vi "TensorFLow.vi"(8 "error in (no error)":errorcluster, 11 "TFinfo In":T1) -> (0 "Label":string, 1 "Percentages":u8[](array[slide]) scale=0.0..100.0, 2 "Fits":dbl[][](array[numeric]), 3 "TFinfo out":T1, 5 "Labels":string)   [LabVIEW 2019]
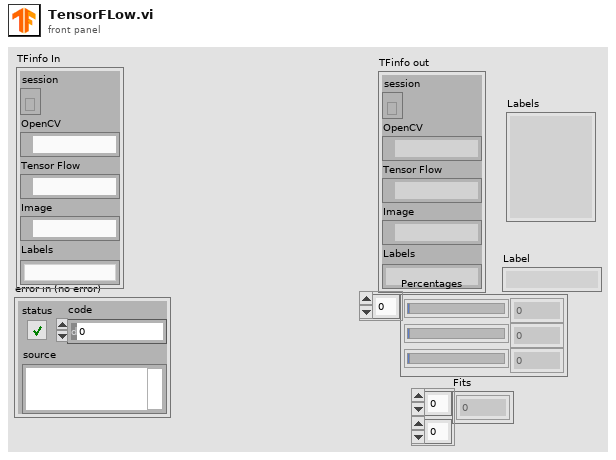
[diagram p1: front panel]
types:
  T1 = cluster{"session":refnum<k35>, "OpenCV":path, "Tensor Flow":path, "Image":path, "Labels":string}
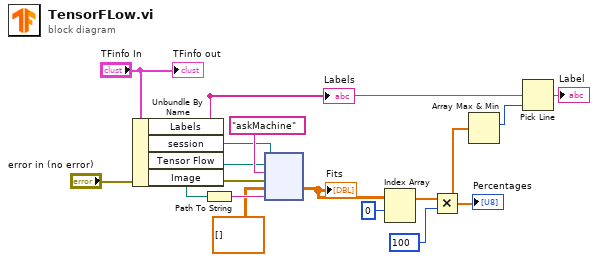
[diagram p0: block diagram]
diagram:
  n1 = Unbundle By Name("TFinfo In") -> ("Labels"=w3:string, "session"=w12:refnum<k35>, "Tensor Flow"=w11:path, "Image"=w9:path)
  "Labels" <- w3
  n2 = Path To String(path=w9) -> (string=w16:string)
  n3 = node(w12, w11, "askMachine" ("function name"), "error in (no error)", dbl[][] [], w16) -> (w8:dbl[][])  [unwired: 1 in, 4 out]
  "Fits" <- w8
  n4 = Index Array(array=w8, index (row)=0) -> (element=w6:dbl[])  [unwired: 1 in]
  n5 = Multiply(x=w6, y=100) -> (x*y=w4:dbl[])
  "Percentages" <- w4
  n6 = Array Max & Min(array=w4) -> (max index (indices)=w2:i32)  [unwired: 3 out]
  n7 = Pick Line(multi-line string=w3, line index=w2) -> (output string=→"Label":string)  [unwired: 1 in]
  "TFinfo out" <- "TFinfo In"
